vi "test- async-resp for csm loop.vi"(8 "error in (no error)":errorcluster, 11 "TestCase in":refnum<class "testcase-csm loop support.lvclass">) -> (0 "error out":errorcluster, 3 "TestCase out":refnum<class "testcase-csm loop support.lvclass">)   [LabVIEW 2017, in "testcase-csm loop support.lvclass"]
uses:
  testcase-csm loop support.lvclass
  56d4bdba-c2f1-4b55-add1-7a078de9da03.vi
  ea54eaf7-6c78-4206-8259-080cdfbb85de.vi
  src/user.lib/_NEVSTOP/Communicable State Machine(CSM)/AdvanceAPI/CSM - Revert Arguments-Safe String.vi
  src/user.lib/_NEVSTOP/Communicable State Machine(CSM)/AdvanceAPI/CSM - Make String Arguments Safe.vi
  src/user.lib/_NEVSTOP/Communicable State Machine(CSM)/AdvanceAPI/CSM - Break Down Multiple States String.vi
  src/user.lib/_NEVSTOP/Communicable State Machine(CSM)/AdvanceAPI/CSM - Compact Multiple States.vi
  src/user.lib/_NEVSTOP/Communicable State Machine(CSM)/AdvanceAPI/CSM - Keywords.vi
  src/user.lib/_NEVSTOP/Communicable State Machine(CSM)/_Shared/Trim Single-line Text.vi
  <vilib>/addons/_JKI Toolkits/VI Tester/TestCase.llb/TestCase.lvclass
  src/user.lib/_NEVSTOP/Communicable State Machine(CSM)/Communicable State Machine.lvlib
  src/user.lib/_NEVSTOP/Communicable State Machine(CSM)/addons/Loop-Support/CSM Loop Support.lvlib
  C:/Program Files (x86)/National Instruments/LabVIEW 2017/vi.lib/addons/_JKI Toolkits/VI Tester/TestCase.llb/TestCase.lvclass
panel:
  out "Arguments":string
  out "State History 2":string
  out "State History":string
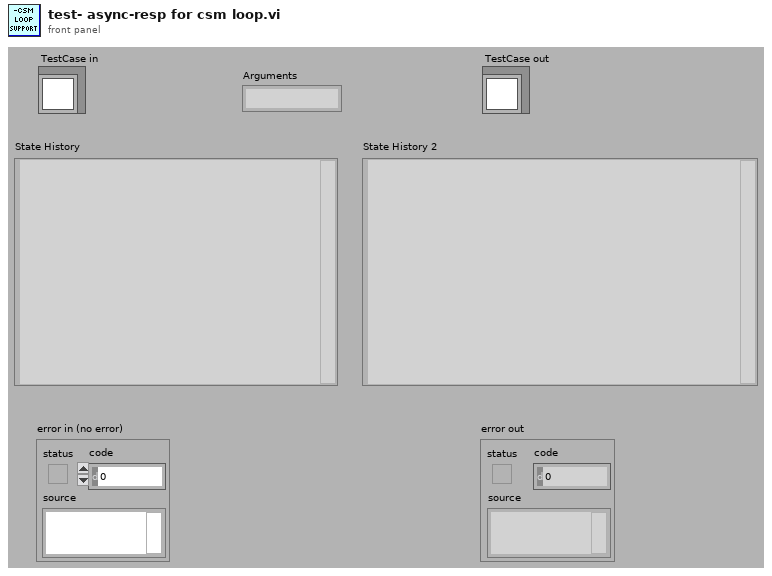
[diagram p1: front panel]
types:
  T1 = enum32{"Invalid", "Standard", "Closed", "Hidden", "Minimized", "Maximized"}
  T2 = enum32{"invalid app kind", "Development System", "Run Time System", "Student Edition", "Embedded LabVIEW", "Evaluation", "Custom"}
  T3 = typedef "Communicable State Machine.lvlib/_CSM_Response Source Message.ctl" = cluster{"‘State":string, "’Arguments":string, "’Error":errorcluster}
  T4 = cluster{"Current VI Reference":refnum<vi>, "Close Panel on Exit?":bool}
  T5 = cluster{"Core":cluster{"Current VI Reference":refnum<vi>, "Close Panel on Exit?":bool}, "diff":dbl, "time":timestamp}
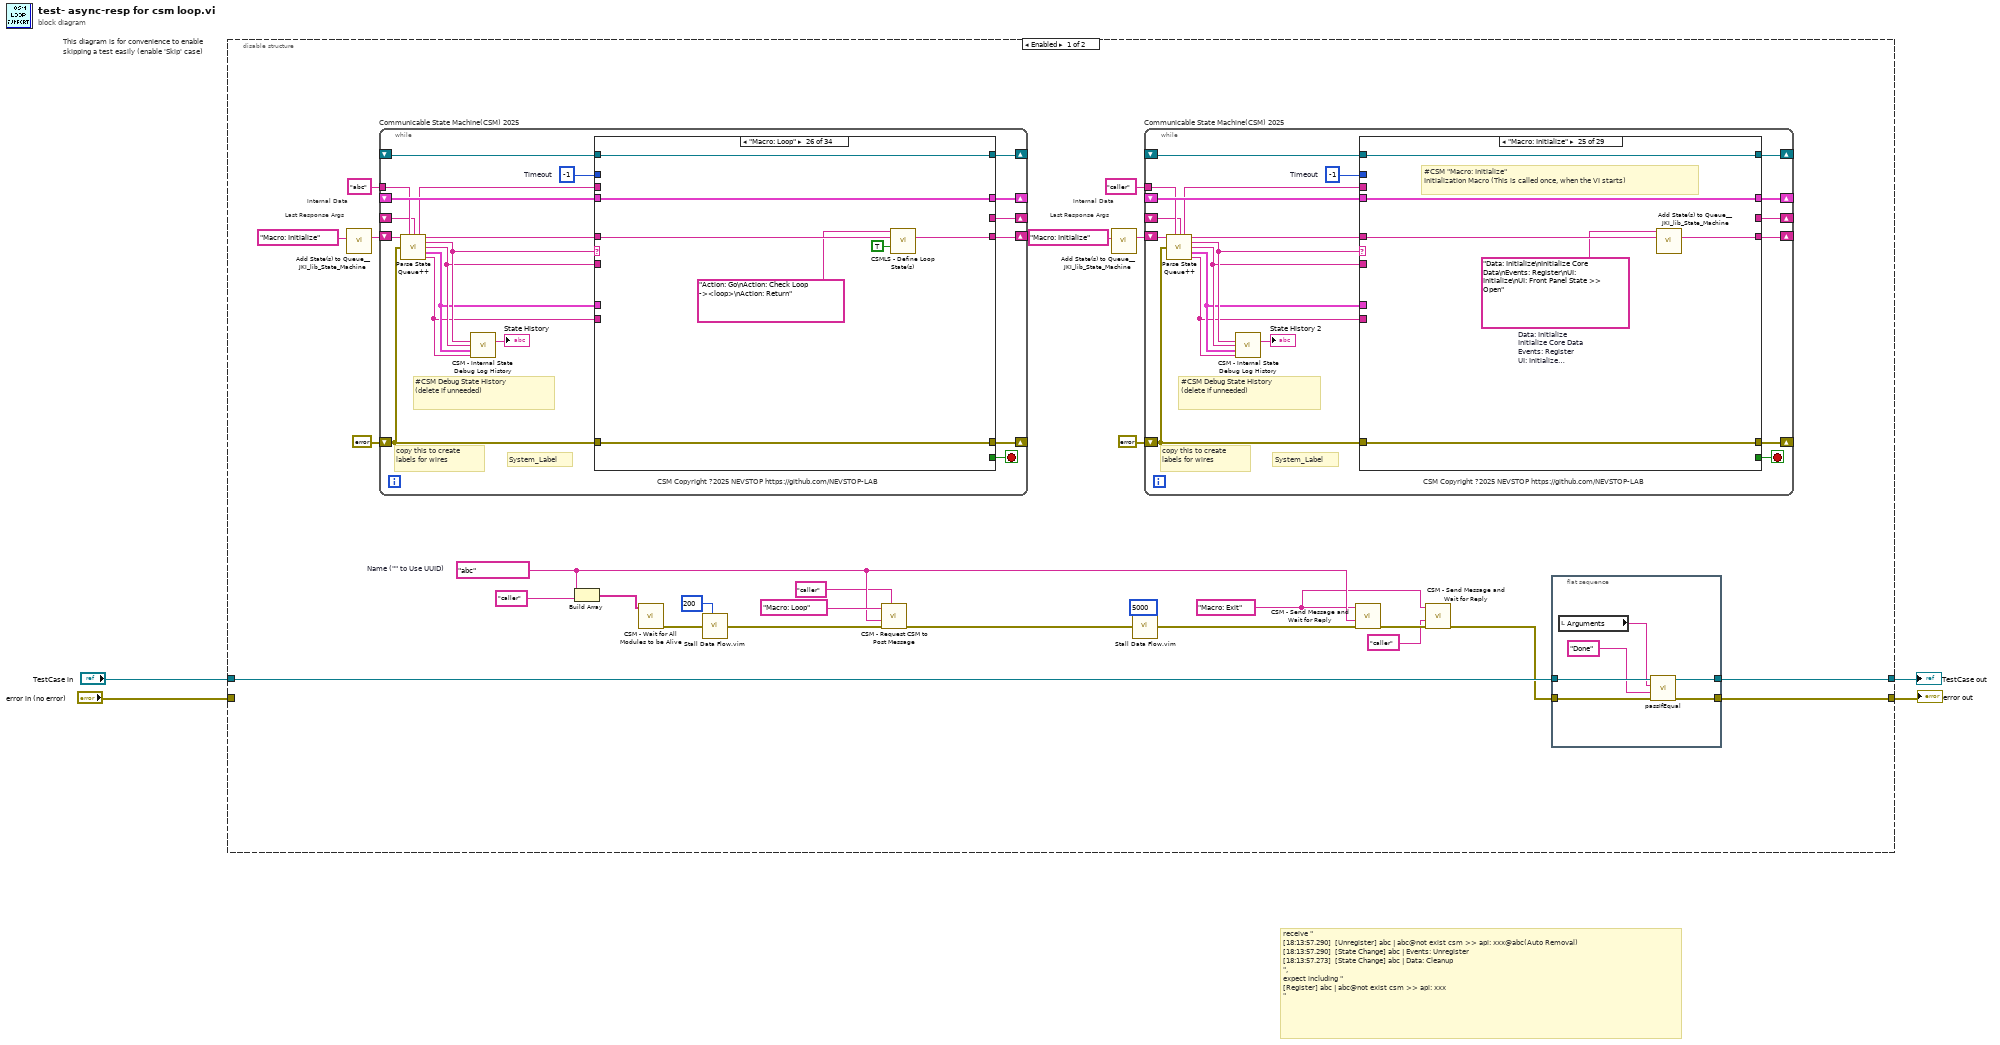
[diagram p0: block diagram]
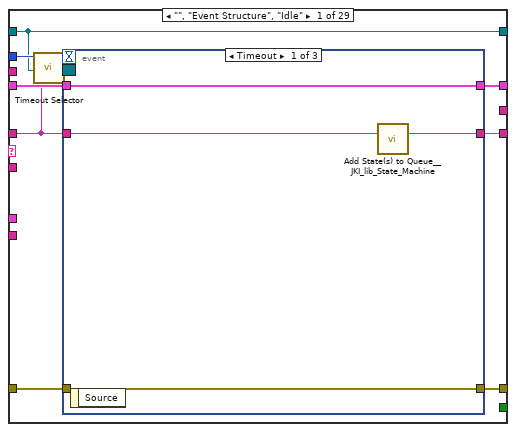
[diagram p2: hidden frame]
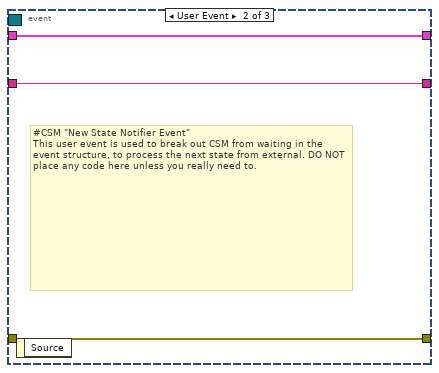
[diagram p3: hidden frame]
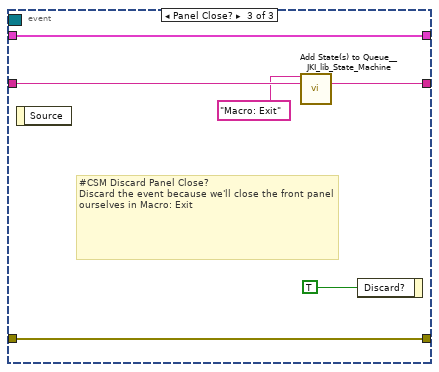
[diagram p4: hidden frame]
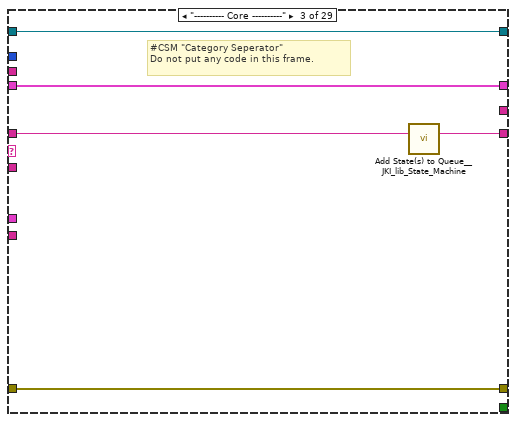
[diagram p6: hidden frame]
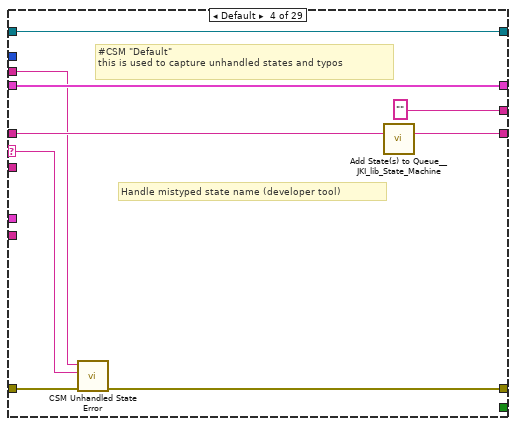
[diagram p7: hidden frame]
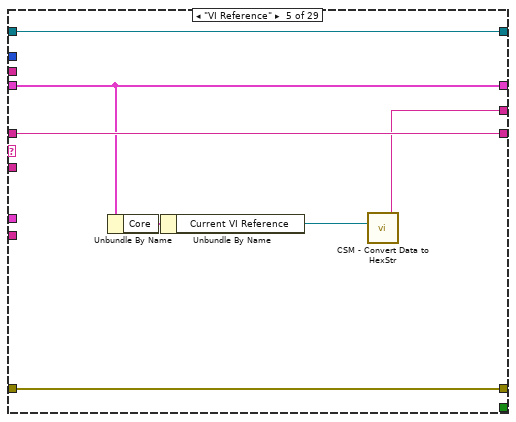
[diagram p8: hidden frame]
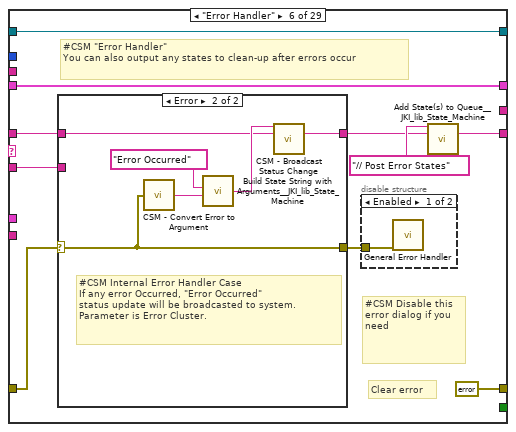
[diagram p9: hidden frame]
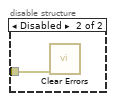
[diagram p10: hidden frame]
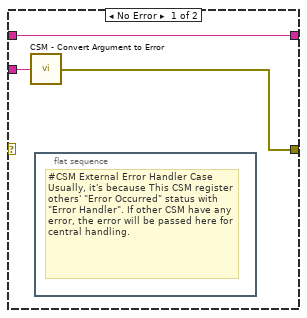
[diagram p11: hidden frame]
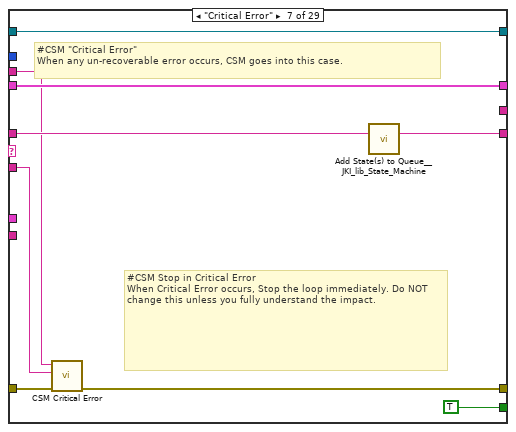
[diagram p12: hidden frame]
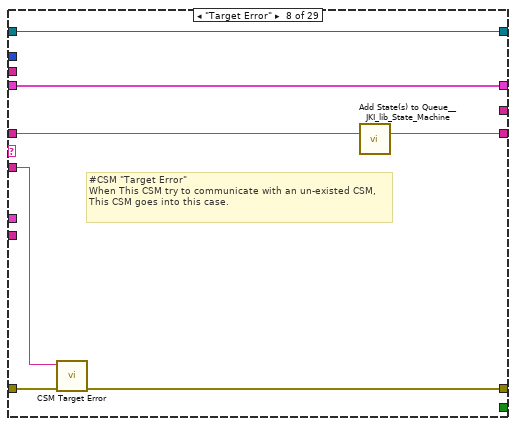
[diagram p13: hidden frame]
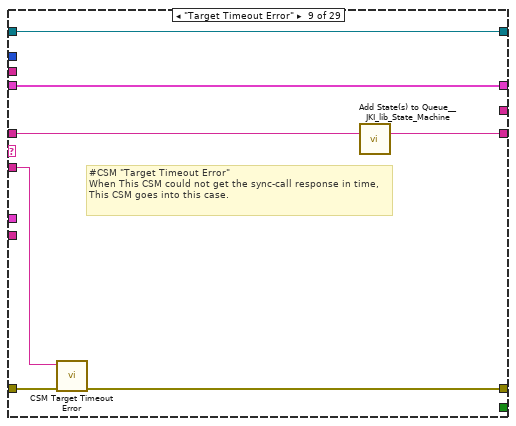
[diagram p14: hidden frame]
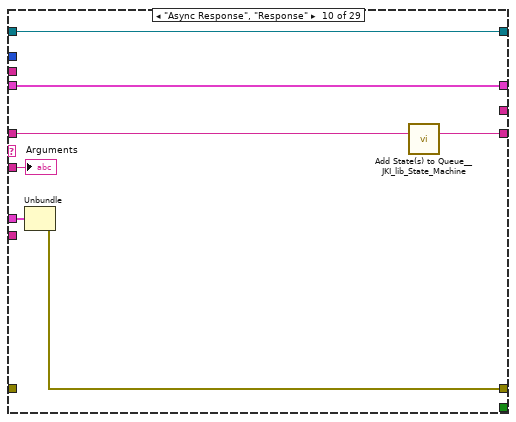
[diagram p15: hidden frame]
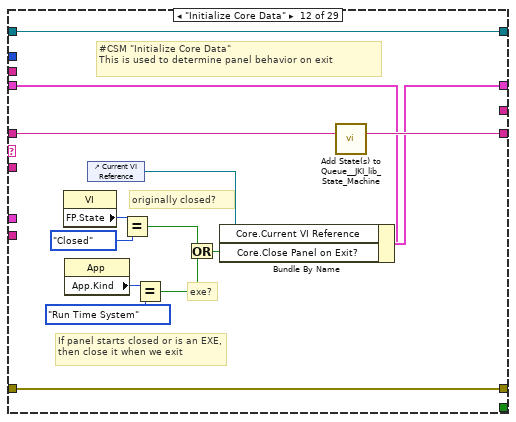
[diagram p17: hidden frame]
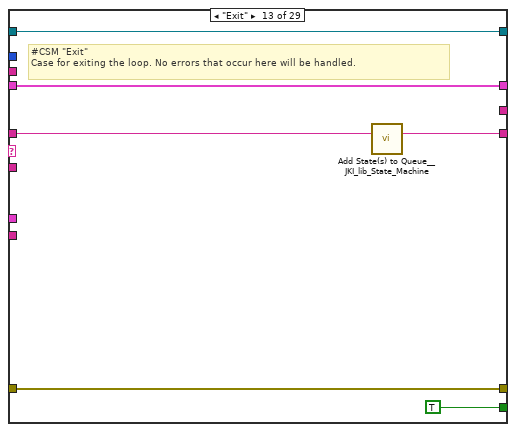
[diagram p18: hidden frame]
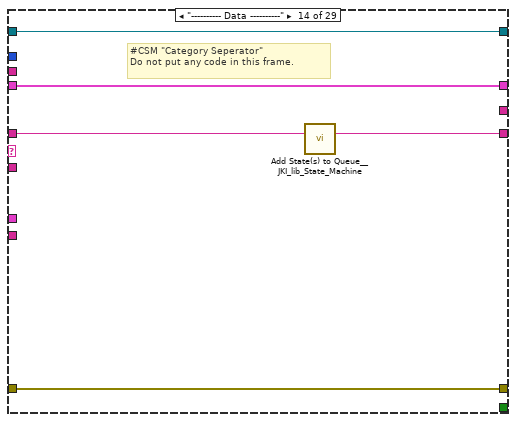
[diagram p19: hidden frame]
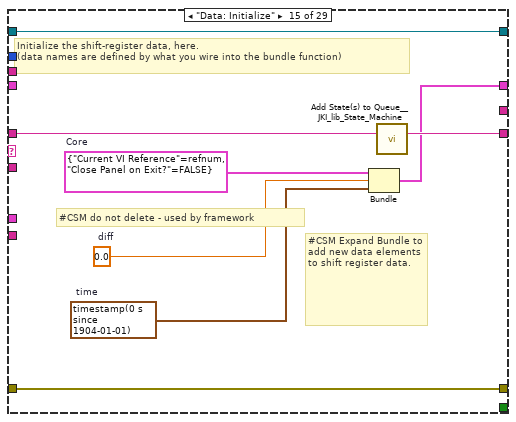
[diagram p20: hidden frame]
diagram:
  # "receive \"\n[18:13:57.290]  [Unregister] abc | abc@not exist csm >> api: xxx@abc(Auto Removal)\n[18:13:57.290]  [State Change] abc | Events: Unregister\n[18:13:57.273]  [State Change] abc | Data: Cleanup\n\", \nexpect including \"\n[Register] abc | abc@not exist csm >> api: xxx\n\""
  n1 = disable-structure "This diagram is for convenience to enable skipping a test easily (enable 'Skip' case)" shown="Enabled" {
    disable-tunnel: "TestCase in" -> [w23 w726]
    disable-tunnel: [w22 w724] -> w1
    disable-tunnel: [w21 w725] -> w3
    disable-tunnel: "error in (no error)" -> [_ w723]
    frame Enabled {
      w7 = "Macro: Exit" ("State")
      w10 = "abc"  # Name ("" to Use UUID)
      # "Last Response Args"
      # "Internal Data"
      # "Last Response Args"
      # "Internal Data"
      n2 = call <vilib>:"Add State(s) to Queue__JKI_lib_State_Machine.vi"("State(s) in (\"\")"="Macro: Initialize" ("Init State(\"Macro: Initialize\")")) -> ("States Out"=w29:string)  [unwired: 14 in]
      n3 = while "Communicable State Machine(CSM) 2025" {
        shift-right: [w369] -> _
        shift-left: _ -> [w368]
        shift-right: [w372] -> _
        shift-left: errorcluster {"status"=FALSE, "code"=0, "source"=""} ("error out") -> [w366]
        shift-right: [w371] -> _
        shift-left: w29 -> [w373]
        tunnel: "abc" ("Name (\"\" to Use UUID)") -> [w362]
        shift-right: [w365] -> _
        shift-left: _ -> [w356]
        shift-right: [w364] -> _
        shift-left: _ -> [w363]
        stop <- w370 stop-if-true
        w367 = -1  # Timeout
        # "#CSM Debug State History\n(delete if unneeded)"
        # "copy this to create labels for wires"
        # "System_Label"
        # "CSM Copyright ?2025 NEVSTOP https://github.com/NEVSTOP-LAB"
        n4 = call "Parse State Queue++.vi"("State Queue"=w373, "Name (\"\" to Use UUID)"=w362, "Response Arguments"=w356, "Previous Error"=w366) -> ("Name Used"=w357:string, "Remaining States"=w374:string, "Current State"=w361:string, "Arguments"=w360:string, "Additional Information"=w359:T3, "Source CSM"=w358:string)  [unwired: 6 in]
        n5 = call "CSM - Internal State Debug Log History.vi"("State"=w361, "Arguments (\"\")"=w360, ">> Response Source Message >>"=w359, "Source (\"\")"=w358) -> ("Debug Log"=→"State History":string)  [unwired: 11 in]
        n6 = case shown="\"Macro: Loop\"" w361 {
          selector: w361 -> [_ _ _ w408 _ _ _ _ _ _ _ _ _ _ _ _ _ _ _ _ _ _ _ _ _ _ _ _ _ _ _ _ w708 _]
          tunnel: w374 -> [w375 w399 w405 w413 w420 w426 w449 w455 w462 w471 w484 w499 w505 w510 w518 w525 w530 w537 w541 w547 w552 w559 w575 w645 w651 w658 w670 w673 w678 w684 w692 w699 w709 w721]
          tunnel: w360 -> [_ _ _ _ _ w425 w444 w454 w461 w470 _ _ _ _ _ _ _ _ _ _ _ w554 w569 _ _ _ _ _ _ w681 _ _ _ _]
          tunnel: w368 -> [w382 w398 w402 w411 w419 w430 w450 w457 w464 w473 w483 w492 w503 w507 _ w520 w527 w536 w540 w544 w550 w557 w571 w642 w648 w655 w667 w672 w677 w683 w689 w696 w705 w719]
          tunnel: [w381 w400 w403 w406 w421 errorcluster {"status"=FALSE, "code"=0, "source"=""} ("error out") w445 w452 w459 w476 w485 w496 w502 w508 w515 w521 w528 w531 w539 w545 w549 w555 w572 w643 w649 w656 w668 w674 w679 w685 w690 w697 w711 w722] -> w372
          tunnel: w366 -> [w380 w400 w403 w414 w421 w427 w451 w453 w460 _ w485 w496 w502 w508 w515 w522 w528 _ w542 w545 w549 w556 w573 w643 w649 w656 w668 w674 w679 w685 w690 w697 w711 w722]
          tunnel: [w383 w399 w404 w412 w420 w422 w448 w458 w465 w472 w484 w498 w504 w509 w517 w524 w529 w537 w541 w546 w551 w558 w574 w644 w650 w657 w669 w673 w678 w684 w691 w698 w712 w721] -> w371
          tunnel: [_ _ _ _ _ _ TRUE _ _ _ _ _ TRUE _ _ _ _ _ _ _ _ _ _ _ _ _ _ _ _ _ _ _ _ _] -> w370
          tunnel: [w379 w398 w402 w411 w419 w430 w450 w457 w464 w474 w483 w497 w503 w507 w516 w520 w527 w536 w540 w544 w550 w557 w571 w642 w648 w655 w667 w672 w677 w683 w689 w694 w701 w719] -> w369
          tunnel: w367 -> [w378 _ _ _ _ _ _ _ _ _ _ _ _ _ _ _ _ _ _ _ _ _ _ _ _ _ _ _ _ _ _ _ _ _]
          tunnel: w358 -> [_ _ _ _ _ _ _ _ _ w468 _ _ _ _ _ _ _ _ _ _ _ _ _ _ _ _ _ _ _ _ _ _ _ _]
          tunnel: w359 -> [_ _ _ _ _ _ _ _ _ w475 _ _ _ _ _ _ _ _ _ _ _ _ _ _ _ _ _ _ _ _ _ _ _ _]
          tunnel: [_ _ _ "" w415 _ _ _ _ _ _ _ _ _ _ _ _ _ _ _ _ _ _ _ _ _ _ _ "API1 Response" w680 _ _ _ "Done" ("HEX String (0-9,A-F)")] -> w365
          tunnel: [w377 w397 w401 w409 w418 w429 w446 w456 w463 w477 w482 w486 w500 w506 w511 w519 w526 w535 w538 w543 w548 w553 w568 w641 w646 w653 w660 w671 w676 w682 w688 w695 w710 w720] -> w364
          tunnel: w363 -> [w377 w397 w401 w409 w418 w429 w446 w456 w463 w477 w482 w486 w500 w506 w511 w519 w526 _ w538 w543 w548 w553 w568 w641 w646 w653 w660 w671 w676 w682 w688 w695 w710 w720]
          tunnel: w357 -> [_ _ _ w407 _ _ w443 _ _ _ _ _ _ _ _ _ _ w534 _ _ _ _ _ _ _ _ _ _ _ _ _ _ _ _]
          frame "", "Event Structure", "Idle" {
            n7 = call "Timeout Selector.vi"("Remaining States"=w375, "Timeout Expected"=w378) -> ("Timeout"=w376:i32)  [unwired: 5 in]
            n8 = event shown="[1] <New State Notifier Event>: User Event" {
              selector: w377 -> [_ _ _]
              dyn-events: _ -> [_ _ _]
              timeout: w376 -> [_ _ _]
              tunnel: w375 -> [w387 w389 w396]
              tunnel: [w386 w389 w395] -> w383
              tunnel: w382 -> [w384 w390 w393]
              tunnel: [w385 w388 w394] -> w381
              tunnel: w380 -> [w385 w388 w394]
              tunnel: [w384 w390 w393] -> w379
              event Timeout {
                n9 = event-data() -> ()  [unwired: 1 in, 1 out]
                n10 = call <vilib>:"Add State(s) to Queue__JKI_lib_State_Machine.vi"("State(s) in (\"\")"=w387) -> ("States Out"=w386:string)  [unwired: 14 in]
              }
              event User Event {
                # "#CSM \"New State Notifier Event\"\nThis user event is used to break out CSM from waiting in the event structure, to process the next state from external. DO NOT place any code here unless you really need to."
                n11 = event-data() -> ()  [unwired: 1 in, 1 out]
              }
              event Panel Close? {
                # "#CSM Discard Panel Close?\nDiscard the event because we'll close the front panel ourselves in Macro: Exit"
                n12 = event-data() -> ()  [unwired: 1 in, 1 out]
                n13 = call <vilib>:"Add State(s) to Queue__JKI_lib_State_Machine.vi"("State(s) in Front (\"\")"="Macro: Exit", "State(s) in (\"\")"=w396) -> ("States Out"=w395:string)  [unwired: 13 in]
                n14 = event-data("Discard?"=TRUE) -> ()  [unwired: 1 in, 1 out]
              }
            }
          }
          frame "CSM Documentation" {
            # "#CSM README FIRST\n\nCommunicable State Machine(CSM) is a LabVIEW application framework that builds upon JKI State Machine(JKISM). It follows the pattern of JKISM and extends the keywords to describe message communication between modules, including concepts such as Sync-Message, Async-Message, Subscription/Unsubscription of status - essential elements for creating reusable code modules. For more information, please visit the CSM wiki: https://nevstop-lab.github.io/CSM-Wiki/\n\nFor instructions on JKI State Machine, visit: http://jki.net/state-machine/\nFor information about CSM, visit: https://github.com/NEVSTOP-LAB"
            # "#CSM \"Documentation\"\nCase for holding CSM Documenation"
          }
          frame "---------- Core ----------" {
            # "#CSM \"Category Seperator\"\nDo not put any code in this frame."
            n15 = call <vilib>:"Add State(s) to Queue__JKI_lib_State_Machine.vi"("State(s) in (\"\")"=w405) -> ("States Out"=w404:string)  [unwired: 14 in]
          }
          frame Default {
            # "#CSM \"Default\"\nthis is used to capture unhandled states and typos"
            # "Handle mistyped state name (developer tool)"
            n16 = call "CSM Unhandled State Error.vi"("error in (no error)"=w414, "Undefined State"=w408, "CSM Name"=w407) -> ("error out"=w406:errorcluster)  [unwired: 8 in]
            n17 = call <vilib>:"Add State(s) to Queue__JKI_lib_State_Machine.vi"("State(s) in (\"\")"=w413) -> ("States Out"=w412:string)  [unwired: 14 in]
          }
          frame "VI Reference" {
            n18 = Unbundle By Name(w419) -> ("Core"=w417:T4)
            n19 = Unbundle By Name(w417) -> ("Current VI Reference"=w416:refnum<vi>)
            n20 = call "CSM - Convert Data to HexStr.vi"("Variant"=w416) -> ("HEX String (0-9,A-F)"=w415:string)  [unwired: 8 in]
          }
          frame "Error Handler" {
            # "#CSM Disable this error dialog if you need"
            # "#CSM \"Error Handler\"\nYou can also output any states to clean-up after errors occur"
            # "Clear error"
            n21 = case shown="Error" w427 {
              selector: w427 -> [_ w437]
              tunnel: [w436 w439] -> w423
              tunnel: w426 -> [w436 w438]
              tunnel: w425 -> [w435 _]
              tunnel: [w434 w437] -> w428
              frame No Error {
                n22 = call "CSM - Convert Argument to Error.vi"("Argument"=w435) -> ("Error"=w434:errorcluster)  [unwired: 4 in]
                n23 = flat-sequence {
                  frame #0 {
                    # "#CSM External Error Handler Case\nUsually, it's because This CSM register others' \"Error Occurred\" status with \"Error Handler\". If other CSM have any error, the error will be passed here for central handling."
                  }
                }
              }
              frame Error {
                # "#CSM Internal Error Handler Case \nIf any error Occurred, \"Error Occurred\" \nstatus update will be broadcasted to system.\nParameter is Error Cluster."
                n24 = call "CSM - Convert Error to Argument.vi"("Error"=w437) -> ("Argument"=w441:string)  [unwired: 4 in]
                n25 = call <vilib>:"Build State String with Arguments__JKI_lib_State_Machine.vi"("Arguments (\"\")"=w441, "State"="Error Occurred" ("Status with Arguments")) -> ("State with Arguments"=w440:string)  [unwired: 4 in]
                n26 = call "CSM - Broadcast Status Change.vi"("Status With Arguments"=w440, "State Queue"=w438) -> ("Remaining States"=w439:string)  [unwired: 13 in]
              }
            }
            n27 = disable-structure shown="Enabled" {
              disable-tunnel: w428 -> [w432 w433]
              frame Enabled {
                n28 = call <vilib>:"General Error Handler.vi"("error in (no error)"=w432) -> ()  [unwired: 10 in, 5 out]
              }
              frame Disabled {
                n29 = call <vilib>:"Clear Errors.vi"("error in (no error)"=w433) -> ()  [unwired: 5 in, 2 out]
              }
            }
            n30 = call <vilib>:"Add State(s) to Queue__JKI_lib_State_Machine.vi"("State(s) in Front (\"\")"="// Post Error States", "State(s) in (\"\")"=w423) -> ("States Out"=w422:string)  [unwired: 13 in]
          }
          frame "Critical Error" {
            # "#CSM Stop in Critical Error\nWhen Critical Error occurs, Stop the loop immediately. Do NOT change this unless you fully understand the impact."
            # "#CSM \"Critical Error\"\nWhen any un-recoverable error occurs, CSM goes into this case."
            n31 = call "CSM Critical Error.vi"("error in (no error)"=w451, "Arugments (As Reason)"=w444, "CSM Name"=w443) -> ("error out"=w445:errorcluster)  [unwired: 8 in]
            n32 = call <vilib>:"Add State(s) to Queue__JKI_lib_State_Machine.vi"("State(s) in (\"\")"=w449) -> ("States Out"=w448:string)  [unwired: 14 in]
          }
          frame "Target Error" {
            # "#CSM \"Target Error\"\nWhen This CSM try to communicate with an un-existed CSM, This CSM goes into this case."
            n33 = call "CSM Target Error.vi"("error in (no error)"=w453, "Arguments (As CSM Name)"=w454) -> ("error out"=w452:errorcluster)  [unwired: 9 in]
            n34 = call <vilib>:"Add State(s) to Queue__JKI_lib_State_Machine.vi"("State(s) in (\"\")"=w455) -> ("States Out"=w458:string)  [unwired: 14 in]
          }
          frame "Target Timeout Error" {
            # "#CSM \"Target Timeout Error\"\nWhen This CSM could not get the sync-call response in time, This CSM goes into this case."
            n35 = call "CSM Target Timeout Error.vi"("error in (no error)"=w460, "Arguments (As CSM Name)"=w461) -> ("error out"=w459:errorcluster)  [unwired: 9 in]
            n36 = call <vilib>:"Add State(s) to Queue__JKI_lib_State_Machine.vi"("State(s) in (\"\")"=w462) -> ("States Out"=w465:string)  [unwired: 14 in]
          }
          frame "Async Response", "Response" {
            n37 = Unbundle(w475) -> ("‘State"=w469:string, "’Arguments"=w467:string, "’Error"=w466:errorcluster)
            n38 = case shown="Default" w469 {
              tunnel: [w481] -> w476
              tunnel: w466 -> [w481]
              tunnel: [w480] -> w474
              tunnel: w473 -> [w480]
              tunnel: [w478] -> w472
              tunnel: w471 -> [w479]
              tunnel: w470 -> [_]
              tunnel: w468 -> [_]
              tunnel: w467 -> [_]
              frame Default {
                # "#CSM Response Comments\nAfter Message is executed, CSM goes to this state for receive the response.\n    For Async Message(->), \"Async Response\" is used. This CSM will goes to \"Async Message Posted\" immediately and receive the \"Async Response\" after the callee finishes the message.\n    For Sync Message(@),  This CSM will wait until the message is done and immediately goes to \"Response\""
                # "#CSM \"Async Response\"\nHandle Async-call Response (\"Async Response\" for ->)"
                # "#CSM \"Response\"\nHandle Sync-call Response (\"Response\" for -@)"
                n39 = call <vilib>:"Add State(s) to Queue__JKI_lib_State_Machine.vi"("State(s) in (\"\")"=w479) -> ("States Out"=w478:string)  [unwired: 14 in]
              }
            }
          }
          frame "Async Message Posted" {
            # "#CSM \"Async Message Posted\"\nAfter Async Message is posted (-> or ->| ), CSM goes to this state for post-action.\nYou can use Argument - State to tell which Async Message is called."
          }
          frame "Initialize Core Data" {
            # "#CSM \"Initialize Core Data\"\nThis is used to determine panel behavior on exit"
            # "originally closed?"
            # "exe?"
            # "If panel starts closed or is an EXE, then close it when we exit"
            n40 = property class="VI"() -> ("FP.State"=w489:T1)  [unwired: 2 in, 2 out]
            n41 = property class="App"() -> ("App.Kind"=w495:T2)  [unwired: 2 in, 2 out]
            n42 = control-ref of="Current VI Reference"() -> (w490:refnum<vi>)
            n43 = Equal?(x=w489, y=T1."Closed" ("Front Panel Window:State")) -> (x = y?=w487:bool)
            n44 = Equal?(x=w495, y=T2."Run Time System" ("Application:Kind")) -> (x = y?=w493:bool)
            n45 = Or(x=w487, y=w493) -> (x .or. y?=w491:bool)
            n46 = Bundle By Name(cluster=w492, "Core.Current VI Reference"=w490, "Core.Close Panel on Exit?"=w491) -> (w497:T5)
            n47 = call <vilib>:"Add State(s) to Queue__JKI_lib_State_Machine.vi"("State(s) in (\"\")"=w499) -> ("States Out"=w498:string)  [unwired: 14 in]
          }
          frame "Exit" {
            # "#CSM \"Exit\"\nCase for exiting the loop. No errors that occur here will be handled."
            n48 = call <vilib>:"Add State(s) to Queue__JKI_lib_State_Machine.vi"("State(s) in (\"\")"=w505) -> ("States Out"=w504:string)  [unwired: 14 in]
          }
          frame "---------- Data ----------" {
            # "#CSM \"Category Seperator\"\nDo not put any code in this frame."
            n49 = call <vilib>:"Add State(s) to Queue__JKI_lib_State_Machine.vi"("State(s) in (\"\")"=w510) -> ("States Out"=w509:string)  [unwired: 14 in]
          }
          frame "Data: Initialize" {
            w512 = T4 {"Current VI Reference"=refnum, "Close Panel on Exit?"=FALSE}  # Core
            w514 = 0.0  # diff
            w513 = timestamp(0 s since 1904-01-01)  # time
            # "#CSM do not delete - used by framework"
            # "#CSM Expand Bundle to add new data elements to shift register data."
            # "Initialize the shift-register data, here.\n(data names are defined by what you wire into the bundle function)"
            n50 = Bundle("Core"=w512, "diff"=w514, "time"=w513) -> (w516:T5)  [unwired: 1 in]
            n51 = call <vilib>:"Add State(s) to Queue__JKI_lib_State_Machine.vi"("State(s) in (\"\")"=w518) -> ("States Out"=w517:string)  [unwired: 14 in]
          }
          frame "Data: Cleanup" {
            # "Cleanup any data and references, here.\n(this is called automatically, by the Macro: Exit)"
            n52 = Unbundle By Name(w520) -> ("Core.Current VI Reference"=w523:refnum<vi>)
            n53 = Close Reference(reference=w523, error in (no error)=w522) -> (error out=w521:errorcluster)
            n54 = call <vilib>:"Add State(s) to Queue__JKI_lib_State_Machine.vi"("State(s) in (\"\")"=w525) -> ("States Out"=w524:string)  [unwired: 14 in]
          }
          frame "---------- Events ----------" {
            # "#CSM \"Category Seperator\"\nDo not put any code in this frame."
            n55 = call <vilib>:"Add State(s) to Queue__JKI_lib_State_Machine.vi"("State(s) in (\"\")"=w530) -> ("States Out"=w529:string)  [unwired: 14 in]
          }
          frame "Events: Register" {
            # "#CSM \"Events: Register\"\nRegister user event. New Message Event is registered to break CSM waiting in event structure by default."
            # "#CSM Register New Message Event\nRegister message event to break Waiting in Event structure."
            n56 = call "CSM - Get New State Notifier Event.vi"("Name (\"\" to Use UUID)"=w534) -> ("error out"=w532:errorcluster, "New State Notifier Event"=w533:refnum<user-event>)  [unwired: 9 in]
            n57 = register-events(error in=w532, w533) -> (reference out=w535:refnum<event-registration>, error out=w531:errorcluster)  [unwired: 1 in]
          }
          frame "Events: Unregister" {
            # "#CSM \"Events: Unregister\"\nUnregister user event."
            n58 = Unregister For Events(event registration refnum=w538, error in=w542) -> (error out=w539:errorcluster)
          }
          frame "---------- UI ----------" {
            # "#CSM \"Category Seperator\"\nDo not put any code in this frame."
            n59 = call <vilib>:"Add State(s) to Queue__JKI_lib_State_Machine.vi"("State(s) in (\"\")"=w547) -> ("States Out"=w546:string)  [unwired: 14 in]
          }
          frame "UI: Initialize" {
            # "#CSM \"UI: Initialize\"\nInitialize the User Interface, here.\n(this is called automatically, by the Macro: Init)"
            n60 = call <vilib>:"Add State(s) to Queue__JKI_lib_State_Machine.vi"("State(s) in (\"\")"=w552) -> ("States Out"=w551:string)  [unwired: 14 in]
          }
          frame "UI: Cursor Set" {
            # "#CSM \"UI: Cursor Set\"\nSet and Unset Cursor Busy.\n(Usage: \"UI: Cursor Set >> Busy|Idle\")"
            # "Argument"
            n61 = disable-structure shown="Default" {
              disable-tunnel: w556 -> [w562 w567]
              disable-tunnel: [w561 w567] -> w555
              disable-tunnel: w554 -> [w560 _]
              frame condition #0 (active) {
                n62 = case shown="\"Idle\", Default" w560 {
                  tunnel: w562 -> [w564 w566]
                  tunnel: [w563 w565] -> w561
                  frame "Idle", Default {
                    n63 = call <vilib>:"Unset Busy.vi"("error in (no error)"=w564) -> ("error out"=w563:errorcluster)  [unwired: 10 in]
                  }
                  frame "Busy" {
                    n64 = call <vilib>:"Set Busy.vi"("error in (no error)"=w566) -> ("error out"=w565:errorcluster)  [unwired: 9 in, 1 out]
                  }
                }
              }
              frame condition #1 {
              }
            }
            n65 = call <vilib>:"Add State(s) to Queue__JKI_lib_State_Machine.vi"("State(s) in (\"\")"=w559) -> ("States Out"=w558:string)  [unwired: 14 in]
          }
          frame "UI: Front Panel State" {
            # "#CSM \"UI: Front Panel State\"\nSet Front Panel Open or Closed\n(Usage: \"UI: Front Panel State >> Open|Close\")"
            # "Argument"
            n66 = Unbundle By Name(w571) -> ("Core.Current VI Reference"=w570:refnum<vi>)
            n67 = call <vilib>:"Add State(s) to Queue__JKI_lib_State_Machine.vi"("State(s) in (\"\")"=w575) -> ("States Out"=w574:string)  [unwired: 14 in]
            n68 = case shown="\"Close\", \"Closed\"" w569 {
              tunnel: w573 -> [w581 w596 w607 w620 w633]
              tunnel: [w583 w597 w609 w622 w635] -> w572
              tunnel: w570 -> [w582 w594 w608 w621 w634]
              frame "Open", "Standard", Default {
                w576 = T1."Standard" ("State")
                n69 = property class="VI"(reference=w582, error in=w581) -> (reference out=w579:refnum<vi>, error out=w580:errorcluster, "FP.State"=w578:T1)
                n70 = Not Equal?(x=w578, y=w576) -> (x != y?=w577:bool)
                n71 = case shown="True" w577 {
                  tunnel: [w587 w589] -> w583
                  tunnel: w580 -> [w586 w589]
                  tunnel: w579 -> [w585 _]
                  tunnel: w576 -> [w584 _]
                  frame True {
                    n72 = invoke class="VI" method="FP.Open"(reference=w585, error in=w586, "Activate"=TRUE, "State"=w584) -> (error out=w587:errorcluster)  [unwired: 1 in, 4 out]
                  }
                  frame False {
                  }
                }
              }
              frame "Close", "Closed" {
                n73 = property class="VI"(reference=w594, error in=w596) -> (reference out=w593:refnum<vi>, error out=w595:errorcluster, "FP.State"=w591:T1)
                n74 = Not Equal?(x=w591, y=T1."Closed" ("Front Panel Window:State")) -> (x != y?=w590:bool)
                n75 = case shown="False" w590 {
                  tunnel: [w598 w601] -> w597
                  tunnel: w595 -> [w598 w600]
                  tunnel: w593 -> [_ w599]
                  frame False {
                  }
                  frame True {
                    n76 = invoke class="VI" method="FP.Close"(reference=w599, error in=w600) -> (error out=w601:errorcluster)  [unwired: 1 in, 2 out]
                  }
                }
              }
              frame "Hidden", "Hide" {
                w602 = T1."Hidden" ("State")
                n77 = property class="VI"(reference=w608, error in=w607) -> (reference out=w605:refnum<vi>, error out=w606:errorcluster, "FP.State"=w604:T1)
                n78 = Not Equal?(x=w604, y=w602) -> (x != y?=w603:bool)
                n79 = case shown="True" w603 {
                  tunnel: [w613 w614] -> w609
                  tunnel: w606 -> [w612 w614]
                  tunnel: w605 -> [w611 _]
                  tunnel: w602 -> [w610 _]
                  frame True {
                    n80 = invoke class="VI" method="FP.Open"(reference=w611, error in=w612, "State"=w610) -> (error out=w613:errorcluster)  [unwired: 2 in, 4 out]
                  }
                  frame False {
                  }
                }
              }
              frame "Minimize", "Minimized" {
                w615 = T1."Minimized" ("State")
                n81 = property class="VI"(reference=w621, error in=w620) -> (reference out=w618:refnum<vi>, error out=w619:errorcluster, "FP.State"=w617:T1)
                n82 = Not Equal?(x=w617, y=w615) -> (x != y?=w616:bool)
                n83 = case shown="True" w616 {
                  tunnel: [w626 w627] -> w622
                  tunnel: w619 -> [w625 w627]
                  tunnel: w618 -> [w624 _]
                  tunnel: w615 -> [w623 _]
                  frame True {
                    n84 = invoke class="VI" method="FP.Open"(reference=w624, error in=w625, "State"=w623) -> (error out=w626:errorcluster)  [unwired: 2 in, 4 out]
                  }
                  frame False {
                  }
                }
              }
              frame "Maximize", "Maximized" {
                w628 = T1."Maximized" ("State")
                n85 = property class="VI"(reference=w634, error in=w633) -> (reference out=w631:refnum<vi>, error out=w632:errorcluster, "FP.State"=w630:T1)
                n86 = Not Equal?(x=w630, y=w628) -> (x != y?=w629:bool)
                n87 = case shown="True" w629 {
                  tunnel: [w639 w640] -> w635
                  tunnel: w632 -> [w638 w640]
                  tunnel: w631 -> [w637 _]
                  tunnel: w628 -> [w636 _]
                  frame True {
                    n88 = invoke class="VI" method="FP.Open"(reference=w637, error in=w638, "State"=w636) -> (error out=w639:errorcluster)  [unwired: 2 in, 4 out]
                  }
                  frame False {
                  }
                }
              }
            }
          }
          frame "---------- Macro ----------" {
            # "#CSM \"Category Seperator\"\nDo not put any code in this frame."
            n89 = call <vilib>:"Add State(s) to Queue__JKI_lib_State_Machine.vi"("State(s) in (\"\")"=w645) -> ("States Out"=w644:string)  [unwired: 14 in]
          }
          frame "Macro: Initialize" {
            w647 = "Data: Initialize\nInitialize Core Data\nEvents: Register\nUI: Initialize\nUI: Front Panel State >> Open"  # Data: Initialize Initialize Core Data Events: Register UI: Initialize UI: Front Panel State >> Open
            # "#CSM \"Macro: Initialize\"\nInitialization Macro (This is called once, when the VI starts)"
            n90 = call <vilib>:"Add State(s) to Queue__JKI_lib_State_Machine.vi"("State(s) in Front (\"\")"=w647, "State(s) in (\"\")"=w651) -> ("States Out"=w650:string)  [unwired: 13 in]
          }
          frame "Macro: Loop" {
            n91 = call "CSMLS - Define Loop State(s).vi"("Loop States"="Action: Go\nAction: Check Loop -><loop>\nAction: Return", "States Queue"=w658, "Add to Front? (F)"=TRUE ("Front(T)/Back(F)")) -> ("Remaining States"=w657:string)  [unwired: 12 in]
          }
          frame "Macro: Exit" {
            # "#CSM \"Macro: Exit\"\nExit Macro (This is called once, when the VI exits)"
            n92 = Unbundle By Name(w667) -> ("Core.Close Panel on Exit?"=w666:bool)
            n93 = Select(t="UI: Front Panel State >> Close", s=w666, f="") -> (s? t:f=w663:string)
            n94 = call <vilib>:"Add State(s) to Queue__JKI_lib_State_Machine.vi"("State(s) in Front (\"\")"="//Exit Sub-Modules ", "State(s) in (\"\")"=w663, "State(s) at Back (\"\")"="Data: Cleanup\nEvents: Unregister\nExit") -> ("States Out"=w661:string)  [unwired: 12 in]
            n95 = call <vilib>:"Add State(s) to Queue__JKI_lib_State_Machine.vi"("State(s) in Front (\"\")"=w661, "State(s) in (\"\")"=w670) -> ("States Out"=w669:string)  [unwired: 13 in]
          }
          frame "---------- API ----------" {
            # "#CSM \"Category Seperator\"\nDo not put any code in this frame."
          }
          frame "API: API1" {
            # "#CSM API Example\nCopy/Rename this case for your own API"
            # "#CSM Response\nConnect this to return the response of your API"
            # "#CSM >> Source CSM >>\nIf you need to tell who triggered this state , use this string. If it's this case itself, this string is \"\"."
            # "#CSM >> Arguments >>\nDeal with the parameter if any"
          }
          frame "API: API2" {
            # "#CSM API Example\nCopy/Rename this case for your own API"
            # "unpack Hex String  to Variant\nif complex parameter is needed."
            n96 = call "CSM - Convert HexStr to Data.vi"("HEX String"=w681) -> ()  [unwired: 7 in, 2 out]
            n97 = disable-structure shown="Disabled" {
              disable-tunnel: [w686 "API2 Response"] -> w680
              frame Disabled {
                # "pack variant to hexstr \nif complex response is needed."
                # "complex Response"
                n98 = call "CSM - Convert Data to HexStr.vi"() -> ("HEX String (0-9,A-F)"=w686:string)  [unwired: 9 in]
              }
              frame Enabled {
              }
            }
          }
          frame "---------- Action ----------" {
            # "#CSM \"Category Seperator\"\nDo not put any code in this frame."
            n99 = call <vilib>:"Add State(s) to Queue__JKI_lib_State_Machine.vi"("State(s) in (\"\")"=w692) -> ("States Out"=w691:string)  [unwired: 14 in]
          }
          frame "Action: Go" {
            n100 = Get Date/Time In Seconds() -> (seconds since 1Jan1904=w693:timestamp)
            n101 = Bundle By Name(cluster=w696, "time"=w693) -> (w694:T5)
            n102 = call <vilib>:"Add State(s) to Queue__JKI_lib_State_Machine.vi"("State(s) in (\"\")"=w699) -> ("States Out"=w698:string)  [unwired: 14 in]
          }
          frame "Action: Check Loop" {
            n103 = Unbundle By Name(w705) -> ("time"=w704:timestamp)
            n104 = Wait (ms)(milliseconds to wait=u32 100) -> ()  [unwired: 1 out]
            n105 = Get Date/Time In Seconds() -> (seconds since 1Jan1904=w706:timestamp)
            n106 = Subtract(x=w706, y=w704) -> (x-y=w700:dbl)
            n107 = Greater?(x=w700, y=3.0) -> (0:w702:bool)
            n108 = case shown="False" w702 {
              tunnel: [w716 w717] -> w712
              tunnel: w709 -> [w715 w717]
              tunnel: w708 -> [w713 _]
              frame False {
                n109 = call "CSMLS - Append Continuous State.vi"("Loop State(s) And Arguments"="" ("Loop State(s) and Arguments"), "Continous State"=w713, "States Queue"=w715) -> ("Remaining States"=w716:string)  [unwired: 8 in]
              }
              frame True {
              }
            }
            n110 = Bundle By Name(cluster=w705, "diff"=w700) -> (w701:T5)
          }
          frame "Action: Return" {
          }
        }
      }
      n111 = Build Array(w10, "caller" ("Name (\"\" to Use UUID)")) -> (w12:string[])
      n112 = call "CSM - Wait for All Modules to be Alive.vi"("CSM Names"=w12) -> ("error out"=w25:errorcluster)  [unwired: 8 in, 2 out]
      n113 = call "Stall Data Flow.vim"("value in"=w25, "milliseconds to wait"=u32 200) -> ("value out"=w18:errorcluster)  [unwired: 1 out]
      n114 = call "CSM - Request CSM to Post Message.vi"("Module Name"="caller" ("Name (\"\" to Use UUID)"), "Error In (No Error)"=w18, "Target Module (\"\" By Default)"=w10, "State"="Macro: Loop") -> ("error out"=w24:errorcluster)  [unwired: 7 in]
      n115 = call <vilib>:"Add State(s) to Queue__JKI_lib_State_Machine.vi"("State(s) in (\"\")"="Macro: Initialize" ("Init State(\"Macro: Initialize\")")) -> ("States Out"=w13:string)  [unwired: 14 in]
      n116 = call "Stall Data Flow.vim"("value in"=w24, "milliseconds to wait"=u32 5000) -> ("value out"=w20:errorcluster)  [unwired: 1 out]
      n117 = while "Communicable State Machine(CSM) 2025" {
        shift-right: [w51] -> _
        shift-left: _ -> [w50]
        shift-right: [w54] -> _
        shift-left: errorcluster {"status"=FALSE, "code"=0, "source"=""} ("error out") -> [w48]
        shift-right: [w53] -> _
        shift-left: w13 -> [w55]
        tunnel: "caller" ("Name (\"\" to Use UUID)") -> [w44]
        shift-right: [w47] -> _
        shift-left: _ -> [w38]
        shift-right: [w46] -> _
        shift-left: _ -> [w45]
        stop <- w52 stop-if-true
        w49 = -1  # Timeout
        # "#CSM Debug State History\n(delete if unneeded)"
        # "copy this to create labels for wires"
        # "System_Label"
        # "CSM Copyright ?2025 NEVSTOP https://github.com/NEVSTOP-LAB"
        n118 = call "Parse State Queue++.vi"("State Queue"=w55, "Name (\"\" to Use UUID)"=w44, "Response Arguments"=w38, "Previous Error"=w48) -> ("Name Used"=w39:string, "Remaining States"=w56:string, "Current State"=w43:string, "Arguments"=w42:string, "Additional Information"=w41:T3, "Source CSM"=w40:string)  [unwired: 6 in]
        n119 = call "CSM - Internal State Debug Log History.vi"("State"=w43, "Arguments (\"\")"=w42, ">> Response Source Message >>"=w41, "Source (\"\")"=w40) -> ("Debug Log"=→"State History 2":string)  [unwired: 11 in]
        n120 = case shown="\"Macro: Initialize\"" w43 {
          selector: w43 -> [_ _ _ w90 _ _ _ _ _ _ _ _ _ _ _ _ _ _ _ _ _ _ _ _ _ _ _ _ _]
          tunnel: w56 -> [w57 w81 w87 w95 w102 w108 w131 w137 w144 w150 w157 w172 w178 w183 w191 w198 w203 w210 w214 w220 w226 w233 w249 w319 w325 w337 w340 w345 w351]
          tunnel: w42 -> [_ _ _ _ _ w107 w126 w136 w143 w148 _ _ _ _ _ _ _ _ _ _ _ w228 w243 _ _ _ _ _ w348]
          tunnel: w50 -> [w64 w80 w84 w93 w101 w112 w132 w139 w146 w152 w156 w165 w176 w180 _ w193 w200 w209 w213 w217 w224 w231 w245 w316 w322 w334 w339 w344 w350]
          tunnel: [w63 w82 w85 w88 w103 errorcluster {"status"=FALSE, "code"=0, "source"=""} ("error out") w127 w134 w141 w149 w158 w169 w175 w181 w188 w194 w201 w204 w212 w218 w223 w229 w246 w317 w323 w335 w341 w346 w352] -> w54
          tunnel: w48 -> [w62 w82 w85 w96 w103 w109 w133 w135 w142 _ w158 w169 w175 w181 w188 w195 w201 _ w215 w218 w223 w230 w247 w317 w323 w335 w341 w346 w352]
          tunnel: [w65 w81 w86 w94 w102 w104 w130 w140 w147 w151 w157 w171 w177 w182 w190 w197 w202 w210 w214 w219 w225 w232 w248 w318 w324 w336 w340 w345 w351] -> w53
          tunnel: [_ _ _ _ _ _ TRUE _ _ _ _ _ TRUE _ _ _ _ _ _ _ _ _ _ _ _ _ _ _ _] -> w52
          tunnel: [w61 w80 w84 w93 w101 w112 w132 w139 w146 w152 w156 w170 w176 w180 w189 w193 w200 w209 w213 w217 w224 w231 w245 w316 w322 w334 w339 w344 w350] -> w51
          tunnel: w49 -> [w60 _ _ _ _ _ _ _ _ _ _ _ _ _ _ _ _ _ _ _ _ _ _ _ _ _ _ _ _]
          tunnel: w40 -> [_ _ _ _ _ _ _ _ _ _ _ _ _ _ _ _ _ _ _ _ _ _ _ _ _ _ _ _ _]
          tunnel: w41 -> [_ _ _ _ _ _ _ _ _ w153 _ _ _ _ _ _ _ _ _ _ _ _ _ _ _ _ _ _ _]
          tunnel: [_ _ _ "" w97 _ _ _ _ _ _ _ _ _ _ _ _ _ _ _ _ _ _ _ _ _ _ "API1 Response" w347] -> w47
          tunnel: [w59 w79 w83 w91 w100 w111 w128 w138 w145 w154 w155 w159 w173 w179 w184 w192 w199 w208 w211 w216 w222 w227 w242 w315 w320 w327 w338 w343 w349] -> w46
          tunnel: w45 -> [w59 w79 w83 w91 w100 w111 w128 w138 w145 w154 w155 w159 w173 w179 w184 w192 w199 _ w211 w216 w222 w227 w242 w315 w320 w327 w338 w343 w349]
          tunnel: w39 -> [_ _ _ w89 _ _ w125 _ _ _ _ _ _ _ _ _ _ w207 _ _ _ _ _ _ _ _ _ _ _]
          frame "", "Event Structure", "Idle" {
            n121 = call "Timeout Selector.vi"("Remaining States"=w57, "Timeout Expected"=w60) -> ("Timeout"=w58:i32)  [unwired: 5 in]
            n122 = event shown="[0] Timeout" {
              selector: w59 -> [_ _ _]
              dyn-events: _ -> [_ _ _]
              timeout: w58 -> [_ _ _]
              tunnel: w57 -> [w69 w71 w78]
              tunnel: [w68 w71 w77] -> w65
              tunnel: w64 -> [w66 w72 w75]
              tunnel: [w67 w70 w76] -> w63
              tunnel: w62 -> [w67 w70 w76]
              tunnel: [w66 w72 w75] -> w61
              event Timeout {
                n123 = event-data() -> ()  [unwired: 1 in, 1 out]
                n124 = call <vilib>:"Add State(s) to Queue__JKI_lib_State_Machine.vi"("State(s) in (\"\")"=w69) -> ("States Out"=w68:string)  [unwired: 14 in]
              }
              event User Event {
                # "#CSM \"New State Notifier Event\"\nThis user event is used to break out CSM from waiting in the event structure, to process the next state from external. DO NOT place any code here unless you really need to."
                n125 = event-data() -> ()  [unwired: 1 in, 1 out]
              }
              event Panel Close? {
                # "#CSM Discard Panel Close?\nDiscard the event because we'll close the front panel ourselves in Macro: Exit"
                n126 = event-data() -> ()  [unwired: 1 in, 1 out]
                n127 = call <vilib>:"Add State(s) to Queue__JKI_lib_State_Machine.vi"("State(s) in Front (\"\")"="Macro: Exit", "State(s) in (\"\")"=w78) -> ("States Out"=w77:string)  [unwired: 13 in]
                n128 = event-data("Discard?"=TRUE) -> ()  [unwired: 1 in, 1 out]
              }
            }
          }
          frame "CSM Documentation" {
            # "#CSM README FIRST\n\nCommunicable State Machine(CSM) is a LabVIEW application framework that builds upon JKI State Machine(JKISM). It follows the pattern of JKISM and extends the keywords to describe message communication between modules, including concepts such as Sync-Message, Async-Message, Subscription/Unsubscription of status - essential elements for creating reusable code modules. For more information, please visit the CSM wiki: https://nevstop-lab.github.io/CSM-Wiki/\n\nFor instructions on JKI State Machine, visit: http://jki.net/state-machine/\nFor information about CSM, visit: https://github.com/NEVSTOP-LAB"
            # "#CSM \"Documentation\"\nCase for holding CSM Documenation"
          }
          frame "---------- Core ----------" {
            # "#CSM \"Category Seperator\"\nDo not put any code in this frame."
            n129 = call <vilib>:"Add State(s) to Queue__JKI_lib_State_Machine.vi"("State(s) in (\"\")"=w87) -> ("States Out"=w86:string)  [unwired: 14 in]
          }
          frame Default {
            # "#CSM \"Default\"\nthis is used to capture unhandled states and typos"
            # "Handle mistyped state name (developer tool)"
            n130 = call "CSM Unhandled State Error.vi"("error in (no error)"=w96, "Undefined State"=w90, "CSM Name"=w89) -> ("error out"=w88:errorcluster)  [unwired: 8 in]
            n131 = call <vilib>:"Add State(s) to Queue__JKI_lib_State_Machine.vi"("State(s) in (\"\")"=w95) -> ("States Out"=w94:string)  [unwired: 14 in]
          }
          frame "VI Reference" {
            n132 = Unbundle By Name(w101) -> ("Core"=w99:T4)
            n133 = Unbundle By Name(w99) -> ("Current VI Reference"=w98:refnum<vi>)
            n134 = call "CSM - Convert Data to HexStr.vi"("Variant"=w98) -> ("HEX String (0-9,A-F)"=w97:string)  [unwired: 8 in]
          }
          frame "Error Handler" {
            # "#CSM Disable this error dialog if you need"
            # "#CSM \"Error Handler\"\nYou can also output any states to clean-up after errors occur"
            # "Clear error"
            n135 = case shown="Error" w109 {
              selector: w109 -> [_ w119]
              tunnel: [w118 w121] -> w105
              tunnel: w108 -> [w118 w120]
              tunnel: w107 -> [w117 _]
              tunnel: [w116 w119] -> w110
              frame No Error {
                n136 = call "CSM - Convert Argument to Error.vi"("Argument"=w117) -> ("Error"=w116:errorcluster)  [unwired: 4 in]
                n137 = flat-sequence {
                  frame #0 {
                    # "#CSM External Error Handler Case\nUsually, it's because This CSM register others' \"Error Occurred\" status with \"Error Handler\". If other CSM have any error, the error will be passed here for central handling."
                  }
                }
              }
              frame Error {
                # "#CSM Internal Error Handler Case \nIf any error Occurred, \"Error Occurred\" \nstatus update will be broadcasted to system.\nParameter is Error Cluster."
                n138 = call "CSM - Convert Error to Argument.vi"("Error"=w119) -> ("Argument"=w123:string)  [unwired: 4 in]
                n139 = call <vilib>:"Build State String with Arguments__JKI_lib_State_Machine.vi"("Arguments (\"\")"=w123, "State"="Error Occurred" ("Status with Arguments")) -> ("State with Arguments"=w122:string)  [unwired: 4 in]
                n140 = call "CSM - Broadcast Status Change.vi"("Status With Arguments"=w122, "State Queue"=w120) -> ("Remaining States"=w121:string)  [unwired: 13 in]
              }
            }
            n141 = disable-structure shown="Enabled" {
              disable-tunnel: w110 -> [w114 w115]
              frame Enabled {
                n142 = call <vilib>:"General Error Handler.vi"("error in (no error)"=w114) -> ()  [unwired: 10 in, 5 out]
              }
              frame Disabled {
                n143 = call <vilib>:"Clear Errors.vi"("error in (no error)"=w115) -> ()  [unwired: 5 in, 2 out]
              }
            }
            n144 = call <vilib>:"Add State(s) to Queue__JKI_lib_State_Machine.vi"("State(s) in Front (\"\")"="// Post Error States", "State(s) in (\"\")"=w105) -> ("States Out"=w104:string)  [unwired: 13 in]
          }
          frame "Critical Error" {
            # "#CSM Stop in Critical Error\nWhen Critical Error occurs, Stop the loop immediately. Do NOT change this unless you fully understand the impact."
            # "#CSM \"Critical Error\"\nWhen any un-recoverable error occurs, CSM goes into this case."
            n145 = call "CSM Critical Error.vi"("error in (no error)"=w133, "Arugments (As Reason)"=w126, "CSM Name"=w125) -> ("error out"=w127:errorcluster)  [unwired: 8 in]
            n146 = call <vilib>:"Add State(s) to Queue__JKI_lib_State_Machine.vi"("State(s) in (\"\")"=w131) -> ("States Out"=w130:string)  [unwired: 14 in]
          }
          frame "Target Error" {
            # "#CSM \"Target Error\"\nWhen This CSM try to communicate with an un-existed CSM, This CSM goes into this case."
            n147 = call "CSM Target Error.vi"("error in (no error)"=w135, "Arguments (As CSM Name)"=w136) -> ("error out"=w134:errorcluster)  [unwired: 9 in]
            n148 = call <vilib>:"Add State(s) to Queue__JKI_lib_State_Machine.vi"("State(s) in (\"\")"=w137) -> ("States Out"=w140:string)  [unwired: 14 in]
          }
          frame "Target Timeout Error" {
            # "#CSM \"Target Timeout Error\"\nWhen This CSM could not get the sync-call response in time, This CSM goes into this case."
            n149 = call "CSM Target Timeout Error.vi"("error in (no error)"=w142, "Arguments (As CSM Name)"=w143) -> ("error out"=w141:errorcluster)  [unwired: 9 in]
            n150 = call <vilib>:"Add State(s) to Queue__JKI_lib_State_Machine.vi"("State(s) in (\"\")"=w144) -> ("States Out"=w147:string)  [unwired: 14 in]
          }
          frame "Async Response", "Response" {
            n151 = Unbundle(w153) -> ("’Error"=w149:errorcluster)  [unwired: 2 out]
            n152 = call <vilib>:"Add State(s) to Queue__JKI_lib_State_Machine.vi"("State(s) in (\"\")"=w150) -> ("States Out"=w151:string)  [unwired: 14 in]
            "Arguments" <- w148
          }
          frame "Async Message Posted" {
            # "#CSM \"Async Message Posted\"\nAfter Async Message is posted (-> or ->| ), CSM goes to this state for post-action.\nYou can use Argument - State to tell which Async Message is called."
          }
          frame "Initialize Core Data" {
            # "#CSM \"Initialize Core Data\"\nThis is used to determine panel behavior on exit"
            # "originally closed?"
            # "exe?"
            # "If panel starts closed or is an EXE, then close it when we exit"
            n153 = property class="VI"() -> ("FP.State"=w162:T1)  [unwired: 2 in, 2 out]
            n154 = property class="App"() -> ("App.Kind"=w168:T2)  [unwired: 2 in, 2 out]
            n155 = control-ref of="Current VI Reference"() -> (w163:refnum<vi>)
            n156 = Equal?(x=w162, y=T1."Closed" ("Front Panel Window:State")) -> (x = y?=w160:bool)
            n157 = Equal?(x=w168, y=T2."Run Time System" ("Application:Kind")) -> (x = y?=w166:bool)
            n158 = Or(x=w160, y=w166) -> (x .or. y?=w164:bool)
            n159 = Bundle By Name(cluster=w165, "Core.Current VI Reference"=w163, "Core.Close Panel on Exit?"=w164) -> (w170:T5)
            n160 = call <vilib>:"Add State(s) to Queue__JKI_lib_State_Machine.vi"("State(s) in (\"\")"=w172) -> ("States Out"=w171:string)  [unwired: 14 in]
          }
          frame "Exit" {
            # "#CSM \"Exit\"\nCase for exiting the loop. No errors that occur here will be handled."
            n161 = call <vilib>:"Add State(s) to Queue__JKI_lib_State_Machine.vi"("State(s) in (\"\")"=w178) -> ("States Out"=w177:string)  [unwired: 14 in]
          }
          frame "---------- Data ----------" {
            # "#CSM \"Category Seperator\"\nDo not put any code in this frame."
            n162 = call <vilib>:"Add State(s) to Queue__JKI_lib_State_Machine.vi"("State(s) in (\"\")"=w183) -> ("States Out"=w182:string)  [unwired: 14 in]
          }
          frame "Data: Initialize" {
            w185 = T4 {"Current VI Reference"=refnum, "Close Panel on Exit?"=FALSE}  # Core
            w187 = 0.0  # diff
            w186 = timestamp(0 s since 1904-01-01)  # time
            # "#CSM do not delete - used by framework"
            # "#CSM Expand Bundle to add new data elements to shift register data."
            # "Initialize the shift-register data, here.\n(data names are defined by what you wire into the bundle function)"
            n163 = Bundle("Core"=w185, "diff"=w187, "time"=w186) -> (w189:T5)  [unwired: 1 in]
            n164 = call <vilib>:"Add State(s) to Queue__JKI_lib_State_Machine.vi"("State(s) in (\"\")"=w191) -> ("States Out"=w190:string)  [unwired: 14 in]
          }
          frame "Data: Cleanup" {
            # "Cleanup any data and references, here.\n(this is called automatically, by the Macro: Exit)"
            n165 = Unbundle By Name(w193) -> ("Core.Current VI Reference"=w196:refnum<vi>)
            n166 = Close Reference(reference=w196, error in (no error)=w195) -> (error out=w194:errorcluster)
            n167 = call <vilib>:"Add State(s) to Queue__JKI_lib_State_Machine.vi"("State(s) in (\"\")"=w198) -> ("States Out"=w197:string)  [unwired: 14 in]
          }
          frame "---------- Events ----------" {
            # "#CSM \"Category Seperator\"\nDo not put any code in this frame."
            n168 = call <vilib>:"Add State(s) to Queue__JKI_lib_State_Machine.vi"("State(s) in (\"\")"=w203) -> ("States Out"=w202:string)  [unwired: 14 in]
          }
          frame "Events: Register" {
            # "#CSM \"Events: Register\"\nRegister user event. New Message Event is registered to break CSM waiting in event structure by default."
            # "#CSM Register New Message Event\nRegister message event to break Waiting in Event structure."
            n169 = call "CSM - Get New State Notifier Event.vi"("Name (\"\" to Use UUID)"=w207) -> ("error out"=w205:errorcluster, "New State Notifier Event"=w206:refnum<user-event>)  [unwired: 9 in]
            n170 = register-events(error in=w205, w206) -> (reference out=w208:refnum<event-registration>, error out=w204:errorcluster)  [unwired: 1 in]
          }
          frame "Events: Unregister" {
            # "#CSM \"Events: Unregister\"\nUnregister user event."
            n171 = Unregister For Events(event registration refnum=w211, error in=w215) -> (error out=w212:errorcluster)
          }
          frame "---------- UI ----------" {
            # "#CSM \"Category Seperator\"\nDo not put any code in this frame."
            n172 = call <vilib>:"Add State(s) to Queue__JKI_lib_State_Machine.vi"("State(s) in (\"\")"=w220) -> ("States Out"=w219:string)  [unwired: 14 in]
          }
          frame "UI: Initialize" {
            # "#CSM \"UI: Initialize\"\nInitialize the User Interface, here.\n(this is called automatically, by the Macro: Init)"
            n173 = call <vilib>:"Add State(s) to Queue__JKI_lib_State_Machine.vi"("State(s) in (\"\")"=w226) -> ("States Out"=w225:string)  [unwired: 14 in]
            n174 = local write "Arguments"("" ("Arguments")) -> ()
          }
          frame "UI: Cursor Set" {
            # "#CSM \"UI: Cursor Set\"\nSet and Unset Cursor Busy.\n(Usage: \"UI: Cursor Set >> Busy|Idle\")"
            # "Argument"
            n175 = disable-structure shown="Default" {
              disable-tunnel: w230 -> [w236 w241]
              disable-tunnel: [w235 w241] -> w229
              disable-tunnel: w228 -> [w234 _]
              frame condition #0 (active) {
                n176 = case shown="\"Idle\", Default" w234 {
                  tunnel: w236 -> [w238 w240]
                  tunnel: [w237 w239] -> w235
                  frame "Idle", Default {
                    n177 = call <vilib>:"Unset Busy.vi"("error in (no error)"=w238) -> ("error out"=w237:errorcluster)  [unwired: 10 in]
                  }
                  frame "Busy" {
                    n178 = call <vilib>:"Set Busy.vi"("error in (no error)"=w240) -> ("error out"=w239:errorcluster)  [unwired: 9 in, 1 out]
                  }
                }
              }
              frame condition #1 {
              }
            }
            n179 = call <vilib>:"Add State(s) to Queue__JKI_lib_State_Machine.vi"("State(s) in (\"\")"=w233) -> ("States Out"=w232:string)  [unwired: 14 in]
          }
          frame "UI: Front Panel State" {
            # "#CSM \"UI: Front Panel State\"\nSet Front Panel Open or Closed\n(Usage: \"UI: Front Panel State >> Open|Close\")"
            # "Argument"
            n180 = Unbundle By Name(w245) -> ("Core.Current VI Reference"=w244:refnum<vi>)
            n181 = call <vilib>:"Add State(s) to Queue__JKI_lib_State_Machine.vi"("State(s) in (\"\")"=w249) -> ("States Out"=w248:string)  [unwired: 14 in]
            n182 = case shown="\"Close\", \"Closed\"" w243 {
              tunnel: w247 -> [w255 w270 w281 w294 w307]
              tunnel: [w257 w271 w283 w296 w309] -> w246
              tunnel: w244 -> [w256 w268 w282 w295 w308]
              frame "Open", "Standard", Default {
                w250 = T1."Standard" ("State")
                n183 = property class="VI"(reference=w256, error in=w255) -> (reference out=w253:refnum<vi>, error out=w254:errorcluster, "FP.State"=w252:T1)
                n184 = Not Equal?(x=w252, y=w250) -> (x != y?=w251:bool)
                n185 = case shown="True" w251 {
                  tunnel: [w261 w263] -> w257
                  tunnel: w254 -> [w260 w263]
                  tunnel: w253 -> [w259 _]
                  tunnel: w250 -> [w258 _]
                  frame True {
                    n186 = invoke class="VI" method="FP.Open"(reference=w259, error in=w260, "Activate"=TRUE, "State"=w258) -> (error out=w261:errorcluster)  [unwired: 1 in, 4 out]
                  }
                  frame False {
                  }
                }
              }
              frame "Close", "Closed" {
                n187 = property class="VI"(reference=w268, error in=w270) -> (reference out=w267:refnum<vi>, error out=w269:errorcluster, "FP.State"=w265:T1)
                n188 = Not Equal?(x=w265, y=T1."Closed" ("Front Panel Window:State")) -> (x != y?=w264:bool)
                n189 = case shown="False" w264 {
                  tunnel: [w272 w275] -> w271
                  tunnel: w269 -> [w272 w274]
                  tunnel: w267 -> [_ w273]
                  frame False {
                  }
                  frame True {
                    n190 = invoke class="VI" method="FP.Close"(reference=w273, error in=w274) -> (error out=w275:errorcluster)  [unwired: 1 in, 2 out]
                  }
                }
              }
              frame "Hidden", "Hide" {
                w276 = T1."Hidden" ("State")
                n191 = property class="VI"(reference=w282, error in=w281) -> (reference out=w279:refnum<vi>, error out=w280:errorcluster, "FP.State"=w278:T1)
                n192 = Not Equal?(x=w278, y=w276) -> (x != y?=w277:bool)
                n193 = case shown="True" w277 {
                  tunnel: [w287 w288] -> w283
                  tunnel: w280 -> [w286 w288]
                  tunnel: w279 -> [w285 _]
                  tunnel: w276 -> [w284 _]
                  frame True {
                    n194 = invoke class="VI" method="FP.Open"(reference=w285, error in=w286, "State"=w284) -> (error out=w287:errorcluster)  [unwired: 2 in, 4 out]
                  }
                  frame False {
                  }
                }
              }
              frame "Minimize", "Minimized" {
                w289 = T1."Minimized" ("State")
                n195 = property class="VI"(reference=w295, error in=w294) -> (reference out=w292:refnum<vi>, error out=w293:errorcluster, "FP.State"=w291:T1)
                n196 = Not Equal?(x=w291, y=w289) -> (x != y?=w290:bool)
                n197 = case shown="True" w290 {
                  tunnel: [w300 w301] -> w296
                  tunnel: w293 -> [w299 w301]
                  tunnel: w292 -> [w298 _]
                  tunnel: w289 -> [w297 _]
                  frame True {
                    n198 = invoke class="VI" method="FP.Open"(reference=w298, error in=w299, "State"=w297) -> (error out=w300:errorcluster)  [unwired: 2 in, 4 out]
                  }
                  frame False {
                  }
                }
              }
              frame "Maximize", "Maximized" {
                w302 = T1."Maximized" ("State")
                n199 = property class="VI"(reference=w308, error in=w307) -> (reference out=w305:refnum<vi>, error out=w306:errorcluster, "FP.State"=w304:T1)
                n200 = Not Equal?(x=w304, y=w302) -> (x != y?=w303:bool)
                n201 = case shown="True" w303 {
                  tunnel: [w313 w314] -> w309
                  tunnel: w306 -> [w312 w314]
                  tunnel: w305 -> [w311 _]
                  tunnel: w302 -> [w310 _]
                  frame True {
                    n202 = invoke class="VI" method="FP.Open"(reference=w311, error in=w312, "State"=w310) -> (error out=w313:errorcluster)  [unwired: 2 in, 4 out]
                  }
                  frame False {
                  }
                }
              }
            }
          }
          frame "---------- Macro ----------" {
            # "#CSM \"Category Seperator\"\nDo not put any code in this frame."
            n203 = call <vilib>:"Add State(s) to Queue__JKI_lib_State_Machine.vi"("State(s) in (\"\")"=w319) -> ("States Out"=w318:string)  [unwired: 14 in]
          }
          frame "Macro: Initialize" {
            w321 = "Data: Initialize\nInitialize Core Data\nEvents: Register\nUI: Initialize\nUI: Front Panel State >> Open"  # Data: Initialize Initialize Core Data Events: Register UI: Initialize UI: Front Panel State >> Open
            # "#CSM \"Macro: Initialize\"\nInitialization Macro (This is called once, when the VI starts)"
            n204 = call <vilib>:"Add State(s) to Queue__JKI_lib_State_Machine.vi"("State(s) in Front (\"\")"=w321, "State(s) in (\"\")"=w325) -> ("States Out"=w324:string)  [unwired: 13 in]
          }
          frame "Macro: Exit" {
            # "#CSM \"Macro: Exit\"\nExit Macro (This is called once, when the VI exits)"
            n205 = Unbundle By Name(w334) -> ("Core.Close Panel on Exit?"=w333:bool)
            n206 = Select(t="UI: Front Panel State >> Close", s=w333, f="") -> (s? t:f=w330:string)
            n207 = call <vilib>:"Add State(s) to Queue__JKI_lib_State_Machine.vi"("State(s) in Front (\"\")"="//Exit Sub-Modules ", "State(s) in (\"\")"=w330, "State(s) at Back (\"\")"="Data: Cleanup\nEvents: Unregister\nExit") -> ("States Out"=w328:string)  [unwired: 12 in]
            n208 = call <vilib>:"Add State(s) to Queue__JKI_lib_State_Machine.vi"("State(s) in Front (\"\")"=w328, "State(s) in (\"\")"=w337) -> ("States Out"=w336:string)  [unwired: 13 in]
          }
          frame "---------- API ----------" {
            # "#CSM \"Category Seperator\"\nDo not put any code in this frame."
          }
          frame "API: API1" {
            # "#CSM API Example\nCopy/Rename this case for your own API"
            # "#CSM Response\nConnect this to return the response of your API"
            # "#CSM >> Source CSM >>\nIf you need to tell who triggered this state , use this string. If it's this case itself, this string is \"\"."
            # "#CSM >> Arguments >>\nDeal with the parameter if any"
          }
          frame "API: API2" {
            # "#CSM API Example\nCopy/Rename this case for your own API"
            # "unpack Hex String  to Variant\nif complex parameter is needed."
            n209 = call "CSM - Convert HexStr to Data.vi"("HEX String"=w348) -> ()  [unwired: 7 in, 2 out]
            n210 = disable-structure shown="Disabled" {
              disable-tunnel: [w353 "API2 Response"] -> w347
              frame Disabled {
                # "pack variant to hexstr \nif complex response is needed."
                # "complex Response"
                n211 = call "CSM - Convert Data to HexStr.vi"() -> ("HEX String (0-9,A-F)"=w353:string)  [unwired: 9 in]
              }
              frame Enabled {
              }
            }
          }
        }
      }
      n212 = call "CSM - Send Message and Wait for Reply.vi"("Error In (No Error)"=w20, "Target Module"=w10, "State"=w7) -> ("error out"=w9:errorcluster)  [unwired: 6 in, 2 out]
      n213 = call "CSM - Send Message and Wait for Reply.vi"("Error In (No Error)"=w9, "Target Module"="caller" ("Name (\"\" to Use UUID)"), "State"=w7) -> ("error out"=w8:errorcluster)  [unwired: 6 in, 2 out]
      n214 = flat-sequence {
        tunnel: w23 -> [w36]
        tunnel: [w35] -> w22
        tunnel: [w34] -> w21
        tunnel: w8 -> [w32]
        frame #0 {
          n215 = local read "Arguments"() -> (w31:string)
          n216 = call-dynamic "passIfEqual.vi"("error in (no error)"=w32, "y"="Done" ("HEX String (0-9,A-F)"), "x"=w31, "TestCase in"=w36) -> ("error out"=w34:errorcluster, "TestCase out"=w35:refnum<class "testcase-csm loop support.lvclass">)  [unwired: 6 in]
        }
      }
    }
    frame Disabled {
      # "skip test result while test is under development"
      n217 = call <vilib>:"skip.vi"("error in (no error)"=w723, "TestCase in"=w726) -> ("error out"=w725:errorcluster, "TestCase out"=w724:refnum<class "testcase-csm loop support.lvclass">)  [unwired: 8 in]
    }
  }
  "error out" <- w3
  "TestCase out" <- w1
